vi "getTestList.vi"(8 "error in (no error)":errorcluster, 10 "listaPruebas":refnum<vi>, 11 "Calibrador in":refnum<class "Calibrador.lvclass">) -> (0 "error out":errorcluster, 2 "listaDePruebas":refnum<class "Prueba.lvclass">[](array[class]), 3 "Calibrador out":refnum<class "Calibrador.lvclass">)   [LabVIEW 2019, in "Calibrador.lvclass"]
uses:
  Calibrador.lvclass
  Pruebas/Prueba/Prueba.lvclass
  Calibrador.lvclass/Calibrador.ctl
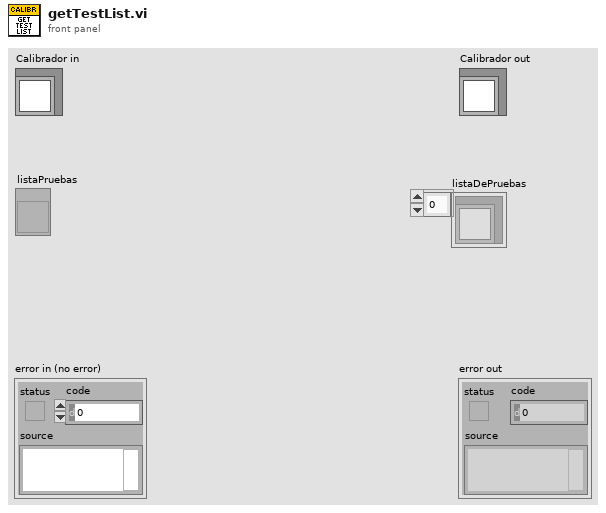
[diagram p1: front panel]
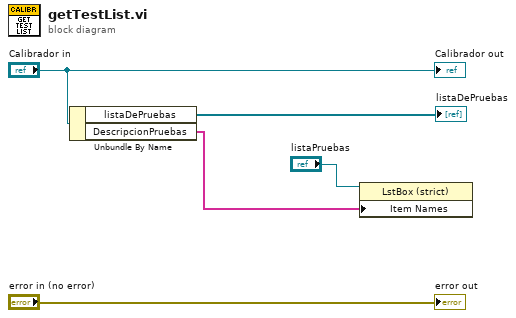
[diagram p0: block diagram]
diagram:
  n1 = Unbundle By Name("Calibrador in") -> ("listaDePruebas"=→"listaDePruebas":refnum<class "Prueba.lvclass">[], "DescripcionPruebas"=w1:string[])
  n2 = property class="LstBox (strict)"(reference="listaPruebas", "Item Names"=w1) -> ()  [unwired: 1 in, 2 out]
  "error out" <- "error in (no error)"
  "Calibrador out" <- "Calibrador in"
